vi "Write Counter Unit.vi"(8 "error in":errorcluster, 10 "Unit":string="ls", 11 "MB_TCP session in":refnum<class "MB_Master_TCP.lvclass">) -> (0 "error out":errorcluster, 3 "MB session out":refnum<class "MB_Master_TCP.lvclass">)   [LabVIEW 2024, in "Bronkhorst Flexi-Flow ModbusTCP API.lvlib"]
uses:
  Bronkhorst Flexi-Flow ModbusTCP API.lvlib
  <vilib>/Plasmionique/MB Master/MB_Master_TCP/MB_Master_TCP.lvclass
  Write String Register.vi
  Read String Register.vi
panel:
  out "Unsigned Char":string
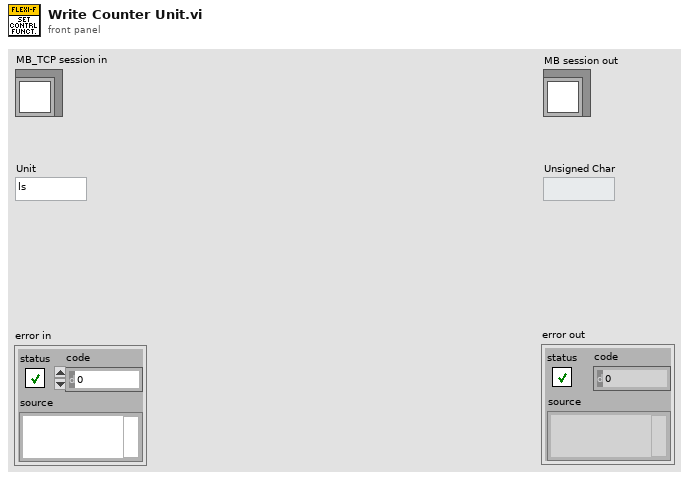
[diagram p1: front panel]
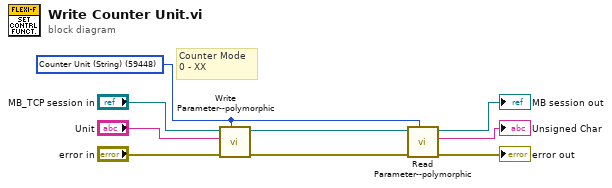
[diagram p0: block diagram]
diagram:
  w1 = u16 59448 items=["Wink"=0, "Control mode"=36, "Alarm mode"=3107, "Alarm setpoint"=3109, "Reset alarm enable"=3113, "Counter unit index"=3330, "Counter setpoint mode"=3333, "Counter mode"=3336, "Reset counter enable"=3337, "Reset"=3688, "Modbus slave address"=4010, "Counter Unit (String)"=59448] ("PDU Address Char 8-bit")
  # "Counter Mode\n0 - XX"
  n1 = call-poly "Write Parameter--polymorphic.vi"("PDU Address String Params"=w1, "error in"="error in", "String"="Unit", "MB_TCP session in"="MB_TCP session in") -> ("error out"=w5:errorcluster, "MB session out"=w7:refnum<class "MB_Master_TCP.lvclass">)  [unwired: 6 in]
  n2 = call-poly "Read Parameter--polymorphic.vi"("PDU Address String Params"=w1, "error in"=w5, "MB_TCP session in"=w7) -> ("error out"=→"error out":errorcluster, "Value"=→"Unsigned Char":string, "MB session out"=→"MB session out":refnum<class "MB_Master_TCP.lvclass">)  [unwired: 6 in]
